vi "Read Variable Core.vi"(8 "error in":errorcluster, 10 "variable name":string, 11 "particle reference in":T1) -> (0 "error out":errorcluster, 2 "variable response":string, 3 "particle reference out":T1)   [LabVIEW 2013, in "Particle API.lvlib"]
uses:
  Particle API.lvlib
  Controls/Particle Reference.ctl
  <vilib>/httpClient/ClientHandle.ctl
  Controls/Device Query JSON.ctl
  <vilib>/httpClient/LabVIEWHTTPClient.lvlib
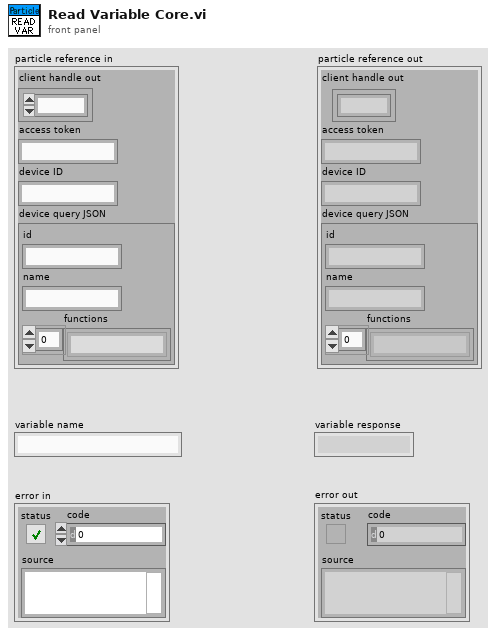
[diagram p1: front panel]
types:
  T1 = typedef "Particle API.lvlib/Particle Reference.ctl" = cluster{"client handle out":T2, "access token":string, "device ID":string, "device query JSON":T3}
  T2 = typedef "LabVIEWHTTPClient.lvlib/ClientHandle.ctl" = refnum<k1>
  T3 = typedef "Particle API.lvlib/Device Query JSON.ctl" = cluster{"id":string, "name":string, "functions":string[]}
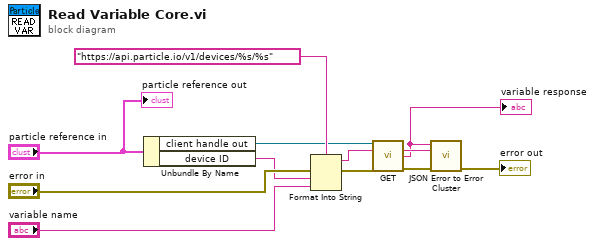
[diagram p0: block diagram]
diagram:
  n1 = Unbundle By Name("particle reference in") -> ("client handle out"=w6:T2, "device ID"=w5:string)
  n2 = Format Into String(format string="https://api.particle.io/v1/devices/%s/%s" ("url"), error in="error in", w5, "variable name") -> (resulting string=w11:string, error out=w7:errorcluster)  [unwired: 1 in]
  n3 = call <vilib>:"GET.vi"("client handle"=w6, "url"=w11, "error in (no error)"=w7) -> ("headers"=w3:string, "body"=w1:string, "error out"=w9:errorcluster)  [unwired: 9 in, 1 out]
  "variable response" <- w1
  n4 = call "JSON Error to Error Cluster.vi"("error in (no error)"=w9, "headers"=w3, "JSON string"=w1) -> ("error out"=→"error out":errorcluster)  [unwired: 8 in]
  "particle reference out" <- "particle reference in"
